vi "Magnetic Sweep 1.0.vi"() -> ()   [LabVIEW 2011]
panel:
  out "Elapsed Time (s) 2":dbl caption="Elapsed Time (s)"
  out "Elapsed Time (s)":dbl
  out "Numeric":i32
  in  "error out":errorcluster
  out "Initial Temperature":string
  out "Zero field reached":bool
  in  "Raw data (ramp down)":path
  in  "Contour plot (ramp down)":path
  out "Target field reached":bool
  out "Temperature":cluster{dbl[], dbl[]}
  out "Resistance":cluster{dbl[], dbl[]}
  out "Magnetic Field":cluster{dbl[], dbl[]}
  in  "Upper limite":dbl
  in  "Temperature\nramping step":dbl
  in  "Heater range":i16(ring) items=["High", "Medium", "Low"]
  in  "D gain":dbl
  in  "I gain":dbl
  in  "P gain":dbl
  in  "Contour plot (ramp up)":path
  out "Time elapsed":string
  in  "Timer":bool caption="Reset"
  in  "date format":enum16{"short", "long", "abbreviated"}(ring)
  in  "Save":bool
  in  "Raw data (ramp  up)":path
  out "Resistance":cluster{dbl[], dbl[]}(graph)
  out "Temperature":cluster{dbl[], dbl[]}(graph)
  out "current time":timestamp
  out "Magnetic\nField":cluster{dbl[], dbl[]}(graph)
  out "Current Resistance":string
  out "Current Temperature":string
  out "Current Field":string
  out "Status":string
  in  "Field Sweep":bool
  in  "Set Parameter":bool
  out "Parameter\nSetup":string
  in  "Ramp rate":dbl
  in  "Traget Field":dbl
  out "Init Response":string
  in  "error in (no error)":errorcluster
  in  "IP Address":string
  in  "Ramp":bool
  in  "Update":bool
  in  "Ramp to Zero":bool
  in  "P Switch":bool
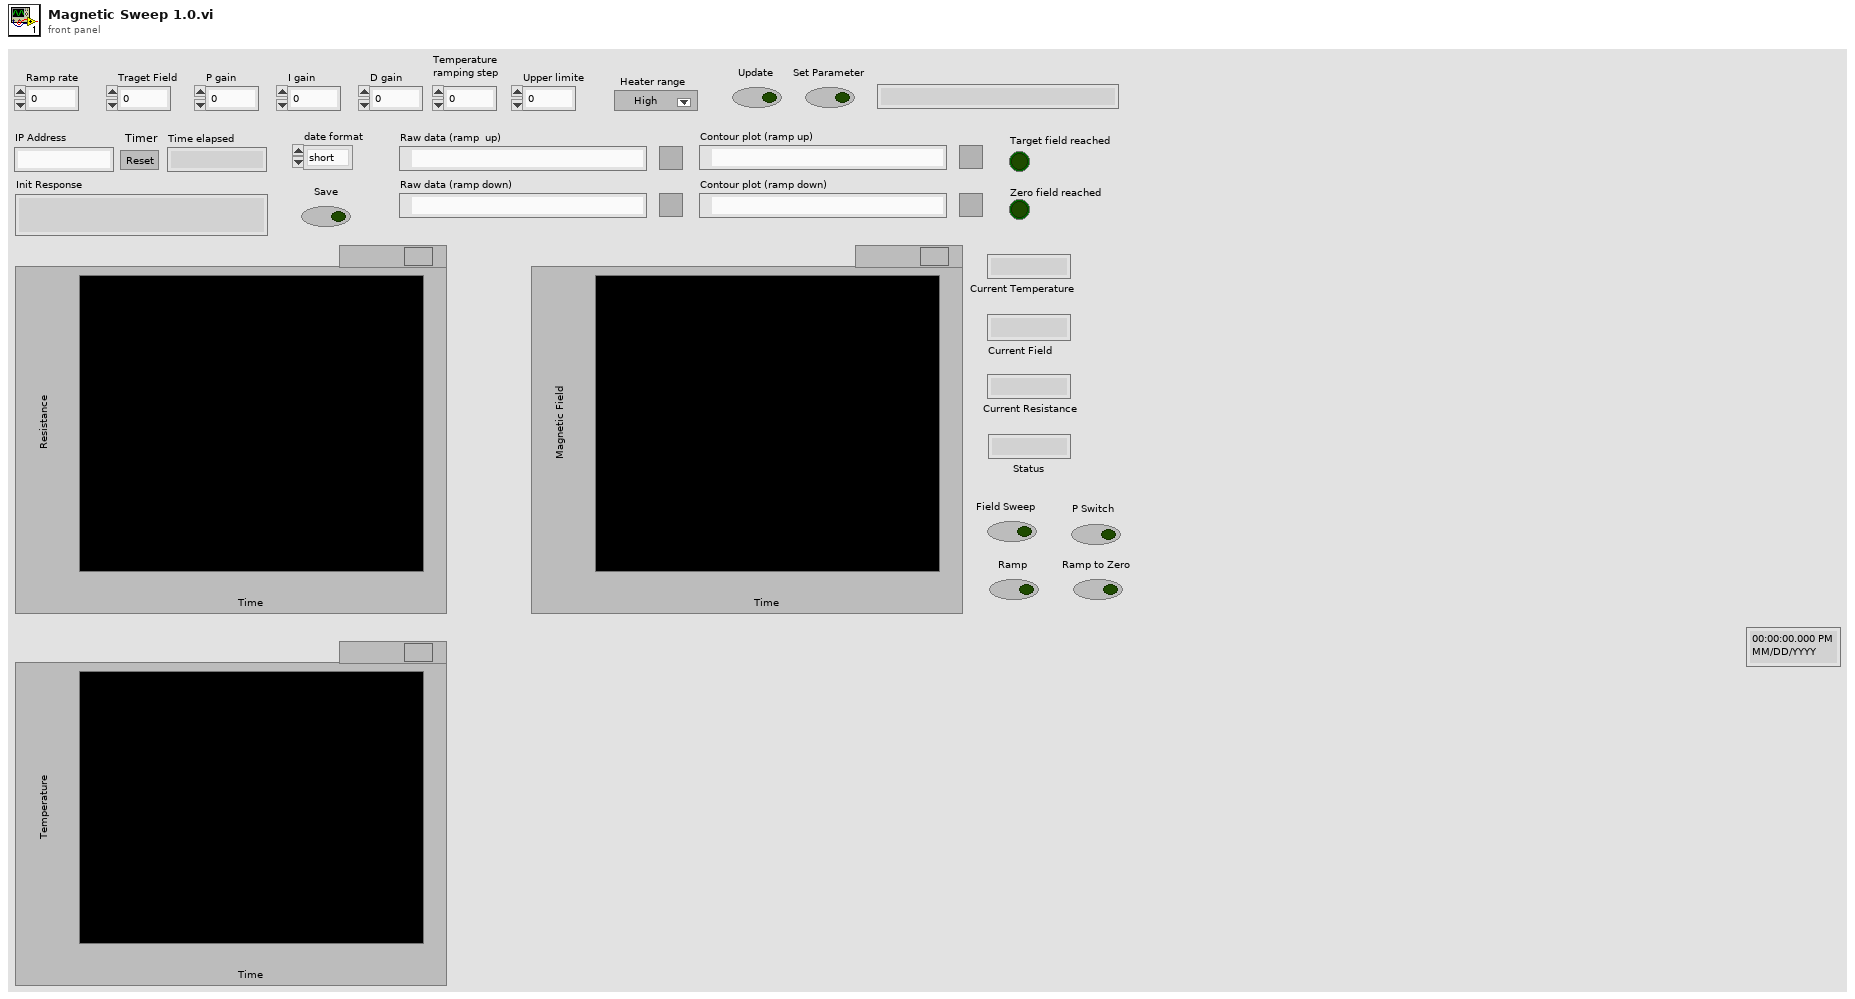
[diagram p1: front panel]
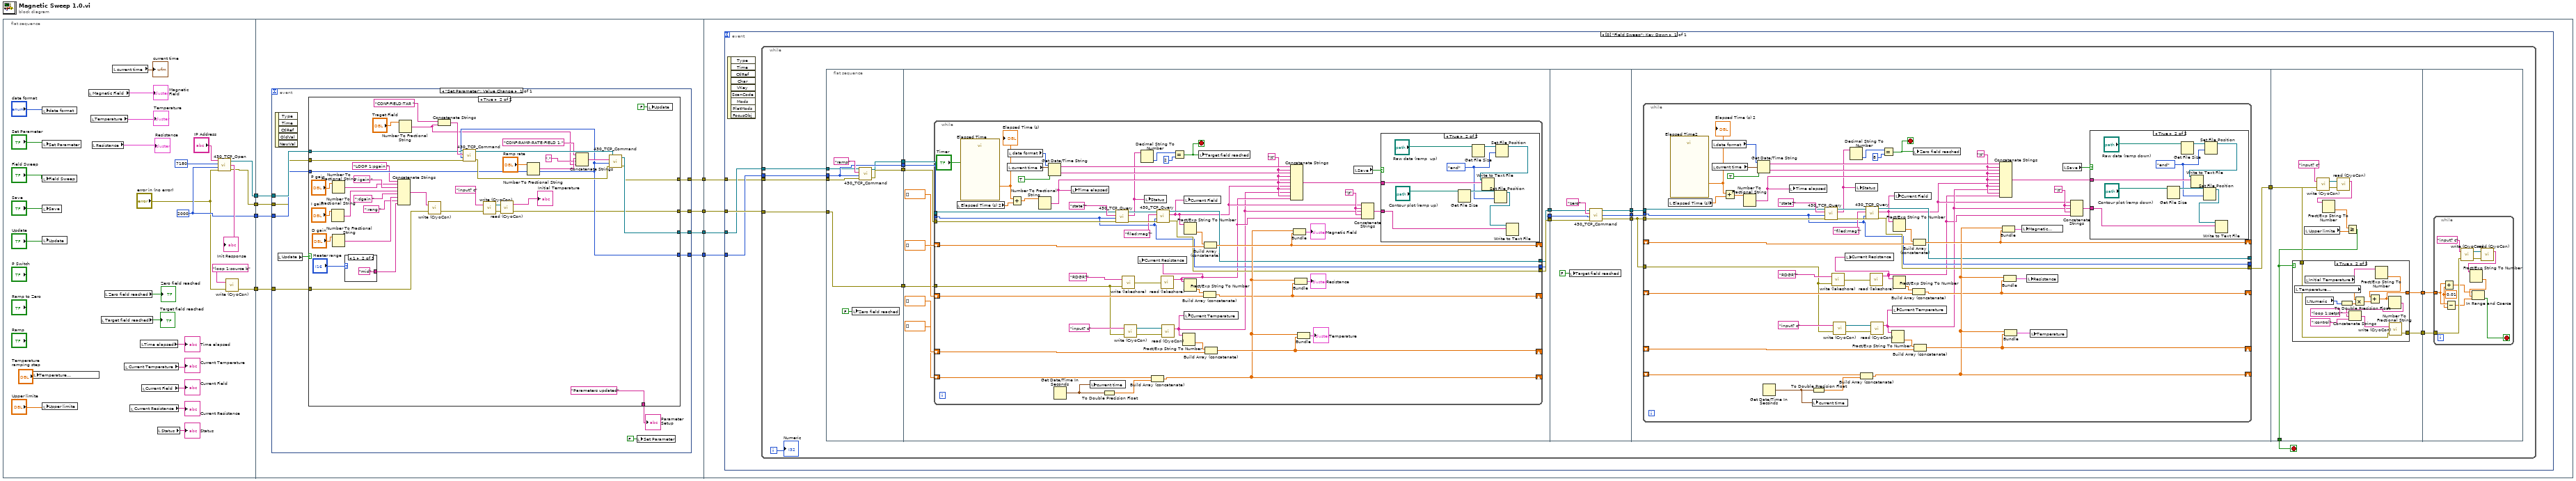
[diagram p0: block diagram]
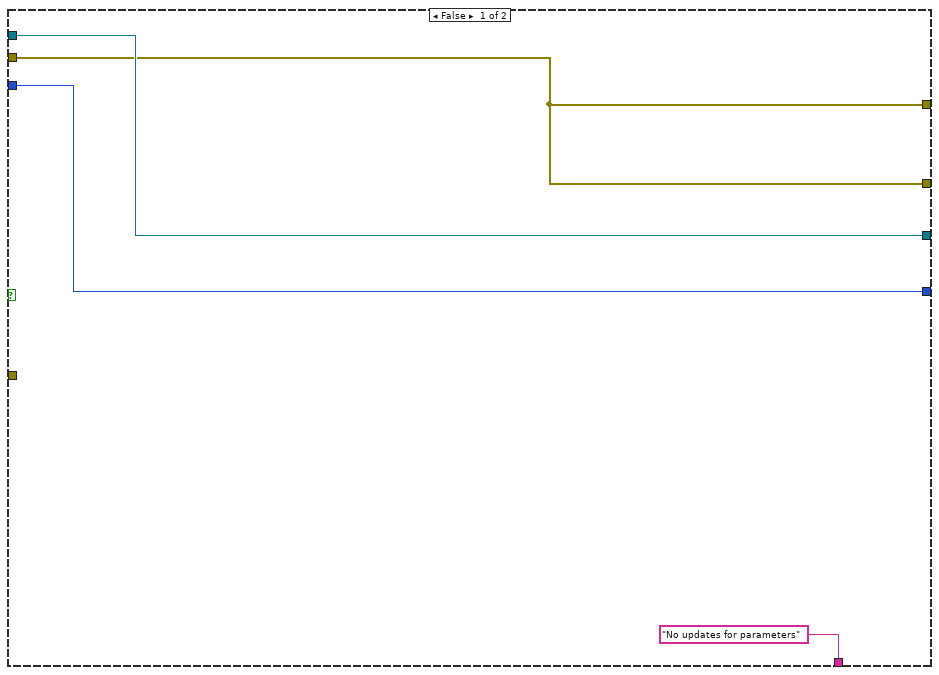
[diagram p2: hidden frame]
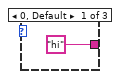
[diagram p3: hidden frame]
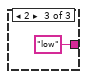
[diagram p4: hidden frame]
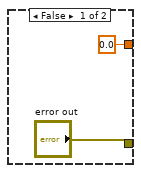
[diagram p7: hidden frame]
diagram:
  n1 = flat-sequence {
    tunnel: [w31] -> w8
    tunnel: [w30] -> w7
    tunnel: [w29] -> w6
    tunnel: [w25] -> w3
    tunnel: w8 -> [w43]
    tunnel: w7 -> [w42]
    tunnel: w6 -> [w41]
    tunnel: [w40] -> w5
    tunnel: [w39] -> w4
    tunnel: w3 -> [w38]
    tunnel: [w37] -> w2
    tunnel: [w36] -> w1
    tunnel: w5 -> [w103]
    tunnel: w4 -> [w102]
    tunnel: w2 -> [w101]
    tunnel: w1 -> [w100]
    frame #0 {
      w30 = 2000 ("Timeout")
      n2 = local write "Temperature\nramping step"("Temperature\nramping step") -> ()
      n3 = local write "date format"("date format") -> ()
      n4 = local write "Set Parameter"("Set Parameter") -> ()
      n5 = local write "Field Sweep"("Field Sweep") -> ()
      n6 = local write "Save"("Save") -> ()
      n7 = local write "Update"("Update") -> ()
      n8 = local write "Upper limite"("Upper limite") -> ()
      n9 = local read "Magnetic Field"() -> (→"Magnetic\nField":cluster{dbl[], dbl[]})
      n10 = local read "Temperature"() -> (→"Temperature":cluster{dbl[], dbl[]})
      n11 = local read "Resistance"() -> (→"Resistance":cluster{dbl[], dbl[]})
      n12 = local read "Target field reached"() -> (→"Target field reached":bool)
      n13 = local read "Zero field reached"() -> (→"Zero field reached":bool)
      n14 = local read "current time"() -> (→"current time":timestamp)
      n15 = local read "Current Temperature"() -> (→"Current Temperature":string)
      n16 = local read "Current Resistance"() -> (→"Current Resistance":string)
      n17 = local read "Time elapsed"() -> (→"Time elapsed":string)
      n18 = local read "Current Field"() -> (→"Current Field":string)
      n19 = local read "Status"() -> (→"Status":string)
      n20 = call "430_TCP_Open.vi"("IP Address"="IP Address", "TCP Port"=7180, "timeout ms (2000)"=w30, "error in (no error)"="error in (no error)") -> ("connection ID"=w31:refnum<k5>, "Init Response"=→"Init Response":string, "error out"=w29:errorcluster)  [unwired: 2 in]
      n21 = call "write (CryoCon).vi"("error in (no error)"="error in (no error)", "write buffer"="loop 1:source b") -> ("error out"=w25:errorcluster)  [unwired: 1 out]
    }
    frame #1 {
      n22 = event shown="[0] \"Set Parameter\": Value Change" {
        selector: _ -> [_]
        dyn-events: _ -> [_]
        timeout: _ -> [_]
        tunnel: w43 -> [w53]
        tunnel: w42 -> [w52]
        tunnel: w41 -> [w51]
        tunnel: [w50] -> w40
        tunnel: [w49] -> w39
        tunnel: w38 -> [w46]
        tunnel: [w45] -> w37
        tunnel: [w44] -> w36
        event "Set Parameter": Value Change {
          n23 = event-data() -> ()  [unwired: 1 in, 5 out]
          n24 = local read "Update"() -> (w54:bool)
          n25 = case shown="True" w54 {
            tunnel: w53 -> [w58 w94]
            tunnel: w52 -> [w57 w84]
            tunnel: w51 -> [w55 w80]
            tunnel: [w58 w85] -> w50
            tunnel: [w57 w84] -> w49
            tunnel: ["No updates for parameters" ("String") "Parameters updated" ("String")] -> w47
            tunnel: w46 -> [_ w69]
            tunnel: [w55 w61] -> w45
            tunnel: [w55 w59] -> w44
            frame False {
            }
            frame True {
              n26 = Number To Fractional String(number="I gain") -> (F-format string=w73:string)  [unwired: 3 in]
              n27 = Number To Fractional String(number="D gain") -> (F-format string=w71:string)  [unwired: 3 in]
              n28 = Number To Fractional String(number="P gain") -> (F-format string=w74:string)  [unwired: 3 in]
              n29 = case shown="1" "Heater range" {
                tunnel: ["hi" "mid" "low"] -> w66
                frame 0, Default {
                }
                frame 1 {
                }
                frame 2 {
                }
              }
              n30 = Concatenate Strings("LOOP 1:pgain " ("write buffer"), w74, ";igain " ("string"), w73, ";dgain " ("string"), w71, ";rang " ("string"), w66) -> (w70:string)
              n31 = Number To Fractional String(number="Traget Field") -> (F-format string=w81:string)  [unwired: 3 in]
              n32 = call "write (CryoCon).vi"("error in (no error)"=w69, "write buffer"=w70) -> ("error out"=w62:errorcluster)  [unwired: 1 out]
              n33 = Concatenate Strings("CONF:FIELD:TAR ", w81) -> (w95:string)
              n34 = call "430_TCP_Command.vi"("error in (no error)"=w80, "Timeout"=w84, "Command"=w95, "connection ID"=w94) -> ("error out"=w93:errorcluster, "connection ID out"=w89:refnum<k5>)  [unwired: 1 out]
              n35 = call "write (CryoCon).vi"("error in (no error)"=w62, "write buffer"="input? c") -> ("error out"=w65:errorcluster, "VISA resource name out"=w64:refnum<visa-resource-name>)
              n36 = call "read (CryoCon).vi"("error in (no error)"=w65, "VISA resource name"=w64) -> ("error out"=w61:errorcluster, "read buffer"=→"Initial Temperature":string)
              n37 = Number To Fractional String(number="Ramp rate") -> (F-format string=w87:string)  [unwired: 3 in]
              n38 = Concatenate Strings("CONF:RAMP:RATE:FIELD 1," ("string"), w87, "," ("string"), w81) -> (w90:string)
              n39 = call "430_TCP_Command.vi"("error in (no error)"=w93, "Timeout"=w84, "Command"=w90, "connection ID"=w89) -> ("error out"=w59:errorcluster, "connection ID out"=w85:refnum<k5>)  [unwired: 1 out]
              n40 = local write "Update"(FALSE ("Update")) -> ()
            }
          }
          "Parameter\nSetup" <- w47
          n41 = local write "Set Parameter"(FALSE ("Set Parameter")) -> ()
        }
      }
    }
    frame #2 {
      n42 = event shown="[0] \"Field Sweep\": Key Down" {
        selector: _ -> [_]
        dyn-events: _ -> [_]
        timeout: _ -> [_]
        tunnel: w103 -> [w106]
        tunnel: w102 -> [w105]
        tunnel: w101 -> [w107]
        tunnel: w100 -> [w104]
        event "Field Sweep": Key Down {
          n43 = event-data() -> ()  [unwired: 1 in, 9 out]
          n44 = while {
            tunnel: w107 -> [w113]
            tunnel: w105 -> [w124]
            tunnel: w106 -> [w122]
            tunnel: w104 -> [w112]
            i -> [w108]
            stop <- w126 stop-if-true
            n45 = flat-sequence {
              tunnel: [w133] -> w125
              tunnel: w124 -> [w132]
              tunnel: [w132] -> w123
              tunnel: w122 -> [w131]
              tunnel: [w130] -> w121
              tunnel: w113 -> [w128]
              tunnel: w112 -> [w129]
              tunnel: [w128] -> w111
              tunnel: w125 -> [w136]
              tunnel: w123 -> [w141]
              tunnel: w121 -> [w140]
              tunnel: [w139] -> w120
              tunnel: [w138] -> w119
              tunnel: [w137] -> w118
              tunnel: w111 -> [w135]
              tunnel: w120 -> [w214]
              tunnel: w119 -> [w213]
              tunnel: w118 -> [w212]
              tunnel: [w211] -> w117
              tunnel: [w210] -> w116
              tunnel: [w209] -> w115
              tunnel: w117 -> [w219]
              tunnel: w116 -> [w218]
              tunnel: w115 -> [w217]
              tunnel: [w216] -> w114
              tunnel: [w284] -> w126
              tunnel: w114 -> [w283]
              tunnel: [w282] -> w110
              tunnel: [w281] -> w109
              tunnel: w110 -> [w308]
              tunnel: w109 -> [w307]
              frame #0 {
                n46 = local write "Zero field reached"(FALSE ("Zero field reached")) -> ()
                n47 = call "430_TCP_Command.vi"("error in (no error)"=w129, "Timeout"=w132, "Command"="ramp", "connection ID"=w131) -> ("error out"=w133:errorcluster, "connection ID out"=w130:refnum<k5>)  [unwired: 1 out]
              }
              frame #1 {
                n48 = while {
                  shift-right: [w181] -> _
                  shift-left: dbl[] [] -> [w186]
                  shift-right: [w180] -> _
                  shift-left: dbl[] [] -> [w191]
                  shift-right: [w178] -> _
                  shift-left: dbl[] [] -> [w188]
                  shift-right: [w179] -> _
                  shift-left: dbl[] [] -> [w182]
                  tunnel: w136 -> [w166]
                  tunnel: w141 -> [w157]
                  tunnel: w140 -> [w165]
                  tunnel: [w159] -> w139
                  tunnel: [w158] -> w138
                  tunnel: [w157] -> w137
                  tunnel: w135 -> [w149]
                  stop <- w160 stop-if-true
                  w170 = "\t"
                  w171 = "\t"
                  n49 = local read "Elapsed Time (s) 2"() -> (w147:dbl)
                  n50 = call "Elapsed Time"("Reset"="Timer") -> ("Elapsed Time (s)"=w148:dbl)  [unwired: 11 in, 7 out]
                  "Elapsed Time (s)" <- w148
                  n51 = local read "current time"() -> (w168:timestamp)
                  n52 = local read "date format"() -> (w151:enum16{"short", "long", "abbreviated"})
                  n53 = Add(x=w148, y=w147) -> (x+y=w146:dbl)
                  n54 = Number To Fractional String(number=w146) -> (F-format string=w156:string)  [unwired: 3 in]
                  n55 = Get Date/Time String(date format (0)=w151, seconds (now)=w168, want seconds? (F)=TRUE) -> (date string=w173:string, time string=w172:string)
                  n56 = Get Date/Time In Seconds() -> (seconds since 1Jan1904=w150:timestamp)
                  n57 = local write "Time elapsed"(w156) -> ()
                  n58 = local write "current time"(w150) -> ()
                  n59 = To Double Precision Float(number=w150) -> (double precision float=w183:dbl)
                  n60 = call "430_TCP_Query.vi"("error in (no error)"=w166, "Timeout"=w157, "Command"="state?", "connection ID"=w165) -> ("error out"=w196:errorcluster, "Response"=w155:string, "connection ID out"=w197:refnum<k5>)  [unwired: 3 in, 2 out]
                  n61 = call "write (lakeshore).vi"("error in (no error)"=w149, "write buffer"="RDGR?") -> ("error out"=w190:errorcluster)
                  n62 = call "write (CryoCon).vi"("error in (no error)"=w149, "write buffer"="input? c") -> ("error out"=w192:errorcluster, "VISA resource name out"=w193:refnum<visa-resource-name>)
                  n63 = Decimal String To Number(string=w155) -> (number=w161:i32)  [unwired: 2 in, 1 out]
                  n64 = local write "Status"(w155) -> ()
                  n65 = Build Array (concatenate)(w182, w183) -> (w179:dbl[])
                  n66 = call "430_TCP_Query.vi"("error in (no error)"=w196, "Timeout"=w157, "Command"="filed:mag?", "connection ID"=w197) -> ("error out"=w159:errorcluster, "Response"=w154:string, "connection ID out"=w158:refnum<k5>)  [unwired: 3 in, 2 out]
                  n67 = call "read (lakeshore).vi"("error in (no error)"=w190) -> ("read buffer"=w153:string)  [unwired: 1 out]
                  n68 = local write "Current Resistance"(w153) -> ()
                  n69 = call "read (CryoCon).vi"("error in (no error)"=w192, "VISA resource name"=w193) -> ("read buffer"=w152:string)  [unwired: 1 out]
                  n70 = Equal?(x=w161, y=2) -> (x = y?=w160:bool)
                  n71 = Fract/Exp String To Number(string=w152) -> (number=w185:dbl)  [unwired: 3 in, 1 out]
                  n72 = Fract/Exp String To Number(string=w153) -> (number=w184:dbl)  [unwired: 3 in, 1 out]
                  n73 = local write "Current Field"(w154) -> ()
                  n74 = Fract/Exp String To Number(string=w154) -> (number=w187:dbl)  [unwired: 3 in, 1 out]
                  n75 = local write "Current Temperature"(w152) -> ()
                  n76 = local write "Target field reached"(w160) -> ()
                  n77 = Build Array (concatenate)(w184, w188) -> (w178:dbl[])
                  n78 = Build Array (concatenate)(w187, w186) -> (w181:dbl[])
                  n79 = Build Array (concatenate)(w185, w191) -> (w180:dbl[])
                  n80 = Concatenate Strings(w173, w171, w172, w171, w156, w171, w154, w171, w152, w171, w153) -> (w176:string)
                  n81 = Bundle(w179, w181) -> (→"Magnetic Field":cluster{dbl[], dbl[]})  [unwired: 1 in]
                  n82 = Bundle(w179, w178) -> (→"Resistance":cluster{dbl[], dbl[]})  [unwired: 1 in]
                  n83 = Bundle(w179, w180) -> (→"Temperature":cluster{dbl[], dbl[]})  [unwired: 1 in]
                  n84 = local read "Save"() -> (w177:bool)
                  n85 = Concatenate Strings(w154, w170, w152, w170, w153) -> (w169:string)
                  n86 = case shown="True" w177 {
                    tunnel: w176 -> [_ w207]
                    tunnel: w169 -> [_ w201]
                    frame False {
                    }
                    frame True {
                      w200 = enum16{"start", "end", "current"}."end" ("from (0:start)")
                      n87 = Get File Size(file="Contour plot (ramp up)") -> (refnum out=w202:refnum<file>)  [unwired: 1 in, 2 out]
                      n88 = Get File Size(file="Raw data (ramp  up)") -> (refnum out=w205:refnum<file>)  [unwired: 1 in, 2 out]
                      n89 = Set File Position(refnum=w202, from (0:start)=w200) -> (refnum out=w199:refnum<file>)  [unwired: 2 in, 1 out]
                      n90 = Set File Position(refnum=w205, from (0:start)=w200) -> (refnum out=w204:refnum<file>)  [unwired: 2 in, 1 out]
                      n91 = Write to Text File(file (use dialog)=w204, text=w207) -> ()  [unwired: 2 in, 3 out]
                      n92 = Write to Text File(file (use dialog)=w199, text=w201) -> ()  [unwired: 2 in, 3 out]
                    }
                  }
                }
              }
              frame #2 {
                n93 = local write "Target field reached"(FALSE ("Target field reached")) -> ()
                n94 = call "430_TCP_Command.vi"("error in (no error)"=w214, "Timeout"=w212, "Command"="zero", "connection ID"=w213) -> ("error out"=w209:errorcluster, "bytes written"=w210:i32, "connection ID out"=w211:refnum<k5>)
              }
              frame #3 {
                n95 = while {
                  shift-right: [w254] -> _
                  shift-left: _ -> [w259]
                  shift-right: [w253] -> _
                  shift-left: _ -> [w264]
                  shift-right: [w251] -> _
                  shift-left: _ -> [w261]
                  shift-right: [w252] -> _
                  shift-left: _ -> [w255]
                  tunnel: w217 -> [w240]
                  tunnel: w217 -> [w241]
                  tunnel: w218 -> [w235]
                  tunnel: w219 -> [w239]
                  tunnel: [w237] -> w216
                  tunnel: [w236] -> _
                  tunnel: [w235] -> _
                  stop <- w223 stop-if-true
                  w244 = "\t"
                  w245 = "\t"
                  n96 = local read "Elapsed Time (s)"() -> (w220:dbl)
                  n97 = call "Elapsed Time2"() -> ("Elapsed Time (s)"=w221:dbl)  [unwired: 12 in, 7 out]
                  "Elapsed Time (s) 2" <- w221
                  n98 = local read "date format"() -> (w224:enum16{"short", "long", "abbreviated"})
                  n99 = local read "current time"() -> (w226:timestamp)
                  n100 = Add(x=w221, y=w220) -> (x+y=w222:dbl)
                  n101 = Number To Fractional String(number=w222) -> (F-format string=w234:string)  [unwired: 3 in]
                  n102 = Get Date/Time String(date format (0)=w224, seconds (now)=w226, want seconds? (F)=TRUE) -> (date string=w247:string, time string=w246:string)
                  n103 = Get Date/Time In Seconds() -> (seconds since 1Jan1904=w225:timestamp)
                  n104 = local write "Time elapsed"(w234) -> ()
                  n105 = local write "current time"(w225) -> ()
                  n106 = To Double Precision Float(number=w225) -> (double precision float=w256:dbl)
                  n107 = call "430_TCP_Query.vi"("error in (no error)"=w241, "Timeout"=w235, "Command"="state?", "connection ID"=w239) -> ("error out"=w269:errorcluster, "Response"=w231:string, "connection ID out"=w270:refnum<k5>)  [unwired: 3 in, 2 out]
                  n108 = call "write (lakeshore).vi"("error in (no error)"=w240, "write buffer"="RDGR?") -> ("error out"=w263:errorcluster)
                  n109 = call "write (CryoCon).vi"("error in (no error)"=w240, "write buffer"="input? c") -> ("error out"=w265:errorcluster, "VISA resource name out"=w266:refnum<visa-resource-name>)
                  n110 = Decimal String To Number(string=w231) -> (number=w238:i32)  [unwired: 2 in, 1 out]
                  n111 = local write "Status"(w231) -> ()
                  n112 = Build Array (concatenate)(w255, w256) -> (w252:dbl[])
                  n113 = call "430_TCP_Query.vi"("error in (no error)"=w269, "Timeout"=w235, "Command"="filed:mag?", "connection ID"=w270) -> ("error out"=w237:errorcluster, "Response"=w232:string, "connection ID out"=w236:refnum<k5>)  [unwired: 3 in, 2 out]
                  n114 = call "read (lakeshore).vi"("error in (no error)"=w263) -> ("read buffer"=w229:string)  [unwired: 1 out]
                  n115 = local write "Current Resistance"(w229) -> ()
                  n116 = call "read (CryoCon).vi"("error in (no error)"=w265, "VISA resource name"=w266) -> ("read buffer"=w233:string)  [unwired: 1 out]
                  n117 = Equal?(x=w238, y=8) -> (x = y?=w223:bool)
                  n118 = Fract/Exp String To Number(string=w233) -> (number=w258:dbl)  [unwired: 3 in, 1 out]
                  n119 = local write "Current Temperature"(w233) -> ()
                  n120 = Fract/Exp String To Number(string=w229) -> (number=w257:dbl)  [unwired: 3 in, 1 out]
                  n121 = Fract/Exp String To Number(string=w232) -> (number=w260:dbl)  [unwired: 3 in, 1 out]
                  n122 = local write "Current Field"(w232) -> ()
                  n123 = Build Array (concatenate)(w257, w261) -> (w251:dbl[])
                  n124 = local write "Zero field reached"(w223) -> ()
                  n125 = Build Array (concatenate)(w260, w259) -> (w254:dbl[])
                  n126 = Build Array (concatenate)(w258, w264) -> (w253:dbl[])
                  n127 = Concatenate Strings(w247, w245, w246, w245, w234, w245, w232, w245, w233, w245, w229) -> (w249:string)
                  n128 = Bundle(w252, w254) -> (w227:cluster{dbl[], dbl[]})  [unwired: 1 in]
                  n129 = Bundle(w252, w251) -> (w230:cluster{dbl[], dbl[]})  [unwired: 1 in]
                  n130 = Bundle(w252, w253) -> (w228:cluster{dbl[], dbl[]})  [unwired: 1 in]
                  n131 = local write "Magnetic\nField"(w227) -> ()
                  n132 = local write "Resistance"(w230) -> ()
                  n133 = local write "Temperature"(w228) -> ()
                  n134 = local read "Save"() -> (w250:bool)
                  n135 = Concatenate Strings(w232, w244, w233, w244, w229) -> (w243:string)
                  n136 = case shown="True" w250 {
                    tunnel: w249 -> [_ w280]
                    tunnel: w243 -> [_ w274]
                    frame False {
                    }
                    frame True {
                      w273 = enum16{"start", "end", "current"}."end" ("from (0:start)")
                      n137 = Get File Size(file="Contour plot (ramp down)") -> (refnum out=w275:refnum<file>)  [unwired: 1 in, 2 out]
                      n138 = Get File Size(file="Raw data (ramp down)") -> (refnum out=w278:refnum<file>)  [unwired: 1 in, 2 out]
                      n139 = Set File Position(refnum=w275, from (0:start)=w273) -> (refnum out=w272:refnum<file>)  [unwired: 2 in, 1 out]
                      n140 = Set File Position(refnum=w278, from (0:start)=w273) -> (refnum out=w277:refnum<file>)  [unwired: 2 in, 1 out]
                      n141 = Write to Text File(file (use dialog)=w277, text=w280) -> ()  [unwired: 2 in, 3 out]
                      n142 = Write to Text File(file (use dialog)=w272, text=w274) -> ()  [unwired: 2 in, 3 out]
                    }
                  }
                }
              }
              frame #4 {
                n143 = local read "Upper limite"() -> (w286:dbl)
                n144 = call "write (CryoCon).vi"("error in (no error)"=w283, "write buffer"="input? c") -> ("error out"=w289:errorcluster, "VISA resource name out"=w290:refnum<visa-resource-name>)
                n145 = call "read (CryoCon).vi"("error in (no error)"=w289, "VISA resource name"=w290) -> ("error out"=w287:errorcluster, "read buffer"=w288:string)
                n146 = Fract/Exp String To Number(string=w288) -> (number=w285:dbl)  [unwired: 3 in, 1 out]
                n147 = Greater Or Equal?(x=w285, y=w286) -> (x >= y?=w284:bool)
                n148 = case shown="True" w284 {
                  tunnel: w287 -> [_ w303]
                  tunnel: ["error out" w300] -> w282
                  tunnel: [0.0 w299] -> w281
                  frame False {
                  }
                  frame True {
                    n149 = local read "Temperature\nramping step"() -> (w297:dbl)
                    n150 = local read "Initial Temperature"() -> (w302:string)
                    n151 = local read "Numeric"() -> (w295:i32)
                    n152 = To Double Precision Float(number=w295) -> (double precision float=w296:dbl)
                    n153 = Multiply(x=w297, y=w296) -> (x*y=w298:dbl)
                    n154 = Fract/Exp String To Number(string=w302) -> (number=w301:dbl)  [unwired: 3 in, 1 out]
                    n155 = Add(x=w301, y=w298) -> (x+y=w299:dbl)
                    n156 = Number To Fractional String(number=w299) -> (F-format string=w304:string)  [unwired: 3 in]
                    n157 = Concatenate Strings("loop 1:setpt " ("write buffer"), w304, ";control" ("string")) -> (w306:string)
                    n158 = call "write (CryoCon).vi"("error in (no error)"=w303, "write buffer"=w306) -> ("error out"=w300:errorcluster)  [unwired: 1 out]
                  }
                }
              }
              frame #5 {
                n159 = while {
                  tunnel: w308 -> [w318]
                  tunnel: w307 -> [w313]
                  stop <- w309 stop-if-true
                  w310 = 0.01 ("y")
                  n160 = Add(x=w313, y=w310) -> (x+y=w312:dbl)
                  n161 = Subtract(x=w313, y=w310) -> (x-y=w311:dbl)
                  n162 = call "write (CryoCon).vi"("error in (no error)"=w318, "write buffer"="input? c") -> ("error out"=w317:errorcluster, "VISA resource name out"=w319:refnum<visa-resource-name>)
                  n163 = call "read (CryoCon).vi"("error in (no error)"=w317, "VISA resource name"=w319) -> ("read buffer"=w315:string)  [unwired: 1 out]
                  n164 = Fract/Exp String To Number(string=w315) -> (number=w314:dbl)  [unwired: 3 in, 1 out]
                  n165 = In Range and Coerce(upper limit=w312, x=w314, lower limit=w311) -> (In Range?=w309:bool)  [unwired: 1 out]
                }
              }
            }
            "Numeric" <- w108
          }
        }
      }
    }
  }
